vi "camera_manual_exp.vi"() -> ()   [LabVIEW 2019]
uses:
  <vilib>/Platform/TimedLoop/XDataNode/timing_clust.ctl
  <vilib>/Platform/TimedLoop/XDataNode/nitl_modes.ctl
  <vilib>/Platform/TimedLoop/XDataNode/wakeup.ctl
  <vilib>/Platform/TimedLoop/XDataNode/XDataNode.xnode
  <vilib>/Platform/TimedLoop/XDataNode/XDNodeRunTimeDep.lvlib
panel:
  out "Stopped":bool=TRUE
  out "Frame Rate":dbl=226.5084075173096
  in  "Analog Control::Gain":dbl=5.0 min=0.0 max=47.994294033026364
  in  "Acquisition Control::Exposure Time":dbl=150.0 min=4.0 max=29999999.0
  in  "Analog Control::Gain Auto":u32(ring) items=["Off", "Once", "Continuous"]
  out "error out":errorcluster
  in  "Acquisition Control::Exposure Auto":u32(ring) items=["Off", "Once", "Continuous"]
  out "?":bool=TRUE
  out "Original Image":T1(plugin-control)
  in  "stop":bool
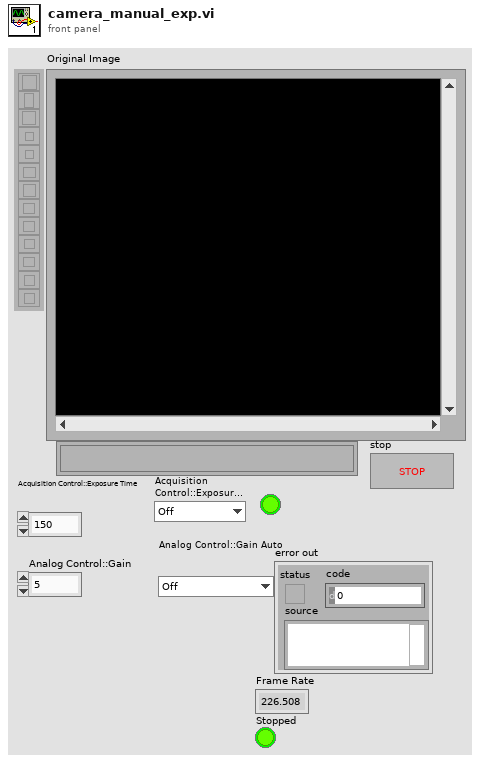
[diagram p1: front panel]
types:
  T1 = typedef "IMAQ Image.ctl" = refnum<image>
  T2 = typedef "XDNodeRunTimeDep.lvlib/timing_clust.ctl" = cluster{"Expected End [f-1]":u64, "Actual End [f-1]":u64, "Finished Late? [f-1]":bool, "Expected End [i-1]":u64, "Actual End [i-1]":u64, "Finished Late? [i-1]":bool, "Expected Start [i]":u64, "Actual Start [i]":u64, "Expected Start [f]":u64, "Actual Start [f]":u64, "Source Name":string, "Structure Name":string, "Period":i64, "Deadline":i64, "Offset":i64, "Start":i64, "Priority":i32, "Timeout":i32, "Mode":T3, "Wakeup Reason":T4, "Error":errorcluster, "Source Type":string, "Secondary Source Type":string, "Global End Time":u64, "Global Start Time":u64, "Frame Duration":u64, "Iteration Duration":u64, "Assigned CPU":i32, "I/O Scan Engine Mode":u32}
  T3 = typedef "XDNodeRunTimeDep.lvlib/nitl_modes.ctl" = enum32{"No Change", "Process missed periods, maintain original phase", "Discard missed periods, maintain original phase", "Process missed periods, ignore original phase", "Discard missed periods, ignore original phase"}
  T4 = typedef "XDNodeRunTimeDep.lvlib/wakeup.ctl" = enum32{"Normal", "Aborted", "Asynchronous wakeup", "Timing source error", "Timed loop error", "Timeout"}
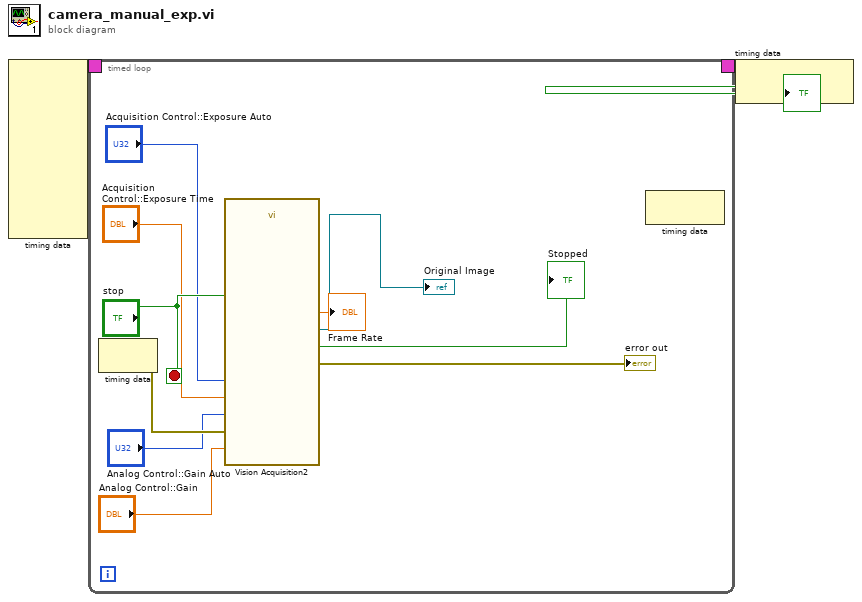
[diagram p0: block diagram]
diagram:
  n1 = node-c288() -> (w3:T2)  [unwired: 10 in]
  n2 = timed-loop {
    timing: w3 -> [_]
    timing-out: [_] -> w2
    stop <- "stop" stop-if-true
    n3 = node-c288() -> (w10:errorcluster)  [unwired: 1 in]
    n4 = call "Vision Acquisition2"("Acquisition Control::Exposure Time"="Acquisition Control::Exposure Time", "Acquisition Control::Exposure Auto"="Acquisition Control::Exposure Auto", "Analog Control::Gain"="Analog Control::Gain", "Analog Control::Gain Auto"="Analog Control::Gain Auto", "Stop (F)"="stop", "error in"=w10) -> ("Image Out"=→"Original Image":T1, "Frame Rate"=→"Frame Rate":dbl, "Stopped"=→"Stopped":bool, "error out"=→"error out":errorcluster)  [unwired: 18 in]
    n5 = node-c288() -> ()  [unwired: 1 in, 1 out]
  }
  n6 = node-c288(w2) -> (→"?":bool)
